vi "RandomishWalk.vi"(0 "Y":dbl, 1 "X":dbl, 2 "Alt Rudder":dbl=10.0, 3 "Default Rudder":dbl=9.0, 4 "Max Radius":dbl=300.0) -> (5 "Velocity":dbl=10.0, 6 "Rudder Command":dbl)   [LabVIEW 2012]
panel:
  in  "Velocity":dbl=10.0
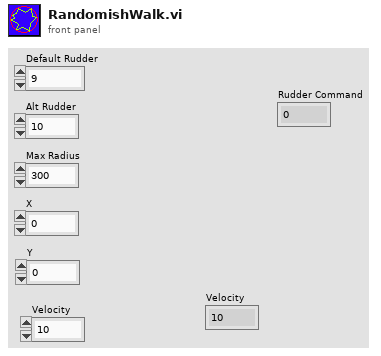
[diagram p1: front panel]
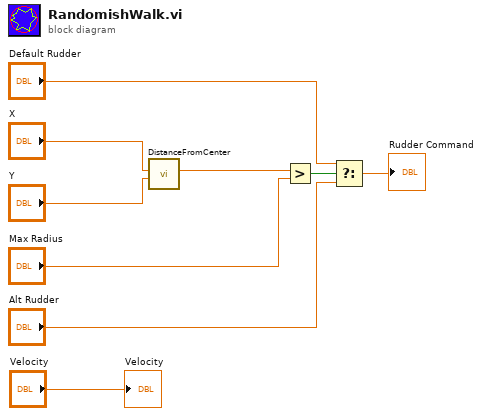
[diagram p0: block diagram]
diagram:
  n1 = call "DistanceFromCenter.vi"("y"="Y", "x"="X") -> ("distance"=w2:dbl)  [unwired: 9 in]
  n2 = Greater?(x=w2, y="Max Radius") -> (0:w7:bool)
  n3 = Select(t="Default Rudder", s=w7, f="Alt Rudder") -> (s? t:f=→"Rudder Command":dbl)
  "Velocity" <- "Velocity"
